vi "Cook Recipe Step.vi"(8 "error in (no error)":errorcluster, 10 "Recipe Step":refnum<class "Recipe Step.lvclass">, 11 "Cooker Actor in":refnum<class "Cooker Actor.lvclass">) -> (0 "error out":errorcluster, 3 "Cooker Actor out":refnum<class "Cooker Actor.lvclass">)   [LabVIEW 2021, in "Cooker Actor.lvlib" / "Cooker Actor.lvclass"]
uses:
  Cooker Actor.lvclass
  Oven Actor/Oven Actor Messages/Apply Heat Msg/Apply Heat Msg.lvclass
  Timer Actor/Timer Actor Messages/Start Count Down Msg/Start Count Down Msg.lvclass
  Support/Recipe Step/Recipe Step.lvclass
  Oven Actor/Oven Actor Messages/Change Oven Type Msg/Change Oven Type Msg.lvclass
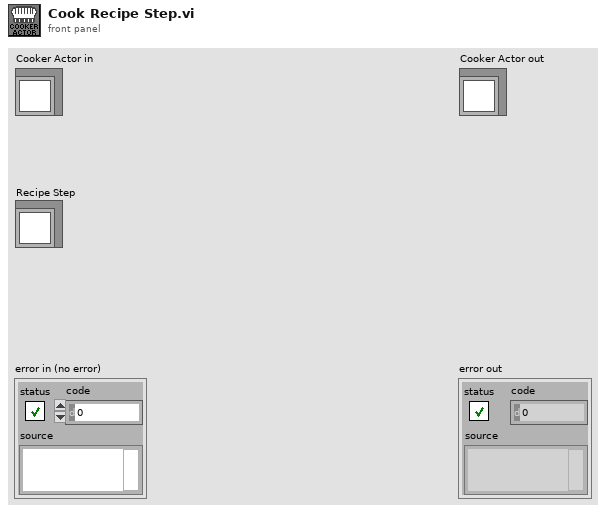
[diagram p1: front panel]
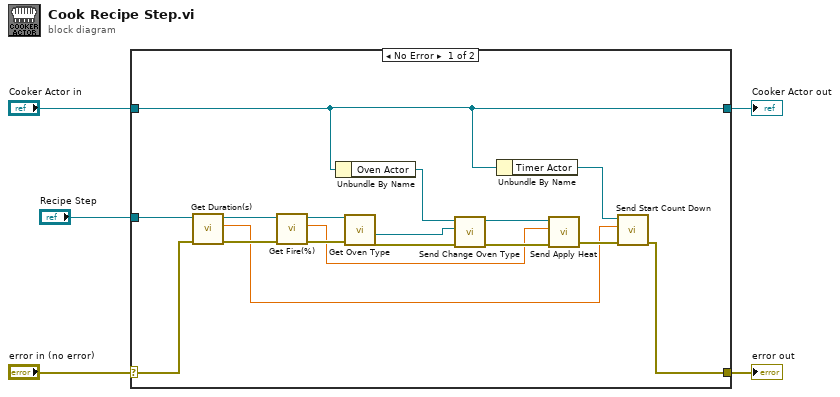
[diagram p0: block diagram]
diagram:
  n1 = case shown="No Error" "error in (no error)" {
    selector: "error in (no error)" -> [w19 w24]
    tunnel: [w18 w24] -> w4
    tunnel: [w17 w23] -> w2
    tunnel: "Cooker Actor in" -> [w17 w23]
    tunnel: "Recipe Step" -> [w20 _]
    frame No Error {
      n2 = call-dynamic "Get Duration(s).vi"("Error In"=w19, "reference in"=w20) -> ("Error Out"=w16:errorcluster, "Duration (s)"=w6:dbl, "reference out"=w15:refnum<class "Recipe Step.lvclass">)  [unwired: 7 in]
      n3 = call-dynamic "Get Fire(%).vi"("Error In"=w16, "reference in"=w15) -> ("Error Out"=w11:errorcluster, "Fire (%)"=w7:dbl, "reference out"=w10:refnum<class "Recipe Step.lvclass">)  [unwired: 7 in]
      n4 = Unbundle By Name(w17) -> ("Oven Actor"=w22:refnum<class "Message Enqueuer.lvclass">)
      n5 = call-dynamic "Get Oven Type.vi"("Error In"=w11, "reference in"=w10) -> ("Error Out"=w9:errorcluster, "Oven Type"=w8:refnum<class "Oven Actor.lvclass">)  [unwired: 6 in, 2 out]
      n6 = call "Send Change Oven Type.vi"("error in (no error)"=w9, "New Oven Type"=w8, "Message Enqueuer"=w22) -> ("error out"=w12:errorcluster, "Message Enqueuer out"=w13:refnum<class "Message Enqueuer.lvclass">)  [unwired: 7 in]
      n7 = Unbundle By Name(w17) -> ("Timer Actor"=w21:refnum<class "Message Enqueuer.lvclass">)
      n8 = call "Send Apply Heat.vi"("error in (no error)"=w12, "Fire (%)"=w7, "Message Enqueuer"=w13) -> ("error out"=w14:errorcluster)  [unwired: 7 in, 1 out]
      n9 = call "Send Start Count Down.vi"("error in (no error)"=w14, "Seconds To Wait"=w6, "Message Enqueuer"=w21) -> ("error out"=w18:errorcluster)  [unwired: 7 in, 1 out]
    }
    frame Error {
    }
  }
  "error out" <- w4
  "Cooker Actor out" <- w2
